vi "Make DS JSON.vi"(9 "Force":bool, 10 "Driverstation prev":T1={"type"="Driverstation", "device"="", "name"="", "data"={">enabled"=FALSE, ">autonomous"=FALSE, ">test"=FALSE, ">estop"=FALSE, ">fms"=FALSE, ">ds"=FALSE, "<match_time"=0.0, ">station"="", ">game_data"=""}}, 11 "Driverstation new":T1={"type"="Driverstation", "device"="", "name"="", "data"={">enabled"=FALSE, ">autonomous"=FALSE, ">test"=FALSE, ">estop"=FALSE, ">fms"=FALSE, ">ds"=FALSE, "<match_time"=0.0, ">station"="", ">game_data"=""}}) -> (3 "delta JSON":string)   [LabVIEW 2019]
uses:
  DS proto.ctl
  DS data proto.ctl
panel:
  out "Complete JSON":string
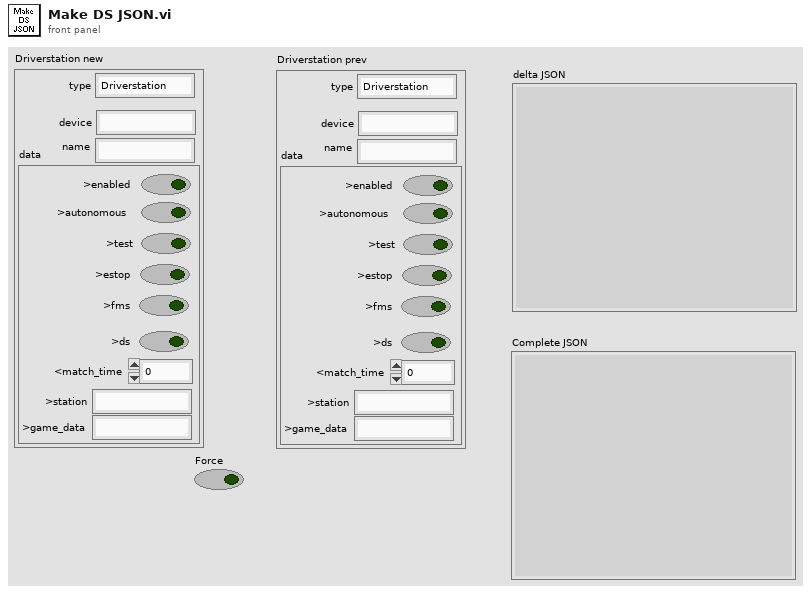
[diagram p1: front panel]
types:
  T1 = typedef "DS proto.ctl" = cluster{"type":string, "device":string, "name":string, "data":T2}
  T2 = typedef "DS data proto.ctl" = cluster{">enabled":bool, ">autonomous":bool, ">test":bool, ">estop":bool, ">fms":bool, ">ds":bool, "<match_time":dbl, ">station":string, ">game_data":string}
  T3 = cluster{"type":bool, "device":bool, "name":bool, "data":cluster{">enabled":bool, ">autonomous":bool, ">test":bool, ">estop":bool, ">fms":bool, ">ds":bool, "<match_time":bool, ">station":bool, ">game_data":bool}}
  T4 = cluster{">enabled":bool, ">autonomous":bool, ">test":bool, ">estop":bool, ">fms":bool, ">ds":bool, "<match_time":bool, ">station":bool, ">game_data":bool}
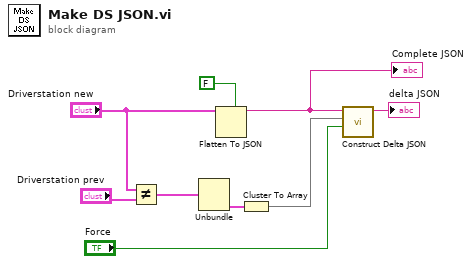
[diagram p0: block diagram]
diagram:
  n1 = Not Equal?(x="Driverstation new", y="Driverstation prev") -> (x != y?=w2:T3)
  n2 = Unbundle(w2) -> ("data"=w6:T4)  [unwired: 3 out]
  n3 = Flatten To JSON(enable LabVIEW extensions? (T)=FALSE, anything="Driverstation new") -> (JSON string=w1:string)  [unwired: 1 in, 1 out]
  "Complete JSON" <- w1
  n4 = Cluster To Array(cluster=w6) -> (array=w4:bool[])
  n5 = call "Construct Delta JSON.vi"("Force"="Force", "Checked Items"=w4, "JSON string"=w1) -> ("Delta JSON"=→"delta JSON":string)  [unwired: 8 in]
